vi "KeyUp.vi"(0 "Virtual Key":T1 items=["LBUTTON"=1, "RBUTTON"=2, "CANCEL"=3, "MBUTTON"=4, "BACKSPACE"=8, "TAB"=9, "CLEAR"=12, "ENTER"=13, "SHIFT"=16, "CTRL"=17, "ALT"=18, "PAUSE"=19, "CAPITAL"=20, "ESCAPE"=27, "SPACE"=32, "PAGEUP"=33, "PAGEDOWN"=34, "END"=35, "HOME"=36, "LEFTARROW"=37, "UPARROW"=38, "RIGHTARROW"=39, "DOWNARROW"=40, "SELECT"=41, "PRINT"=42, "EXECUTE"=43, "PRINTSCREEN"=44, "INSERT"=45, "DELETE"=46, "HELP"=47, "0"=48, "1"=49, "2"=50, "3"=51, "4"=52, "5"=53, "6"=54, "7"=55, "8"=56, "9"=57, "A"=65, "B"=66, "C"=67, "D"=68, "E"=69, "F"=70, "G"=71, "H"=72, "I"=73, "J"=74, "K"=75, "L"=76, "M"=77, "N"=78, "O"=79, "P"=80, "Q"=81, "R"=82, "S"=83, "T"=84, "U"=85, "V"=86, "W"=87, "X"=88, "Y"=89, "Z"=90, "LWIN"=91, "RWIN"=92, "APPS"=93, "NUMPAD0"=96, "NUMPAD1"=97, "NUMPAD2"=98, "NUMPAD3"=99, "NUMPAD4"=100, "NUMPAD5"=101, "NUMPAD6"=102, "NUMPAD7"=103, "NUMPAD8"=104, "NUMPAD9"=105, "MULTIPLY"=106, "ADD"=107, "SEPERATOR"=108, "SUBTRACT"=109, "DECIMAL"=110, "DIVIDE"=111, "F1"=112, "F2"=113, "F3"=114, "F4"=115, "F5"=116, "F6"=117, "F7"=118, "F8"=119, "F9"=120, "F10"=121, "F11"=122, "F12"=123, "F13"=124, "F14"=125, "F15"=126, "F16"=127, "F17"=128, "F18"=129, "F19"=130, "F20"=131, "F21"=132, "F22"=133, "F23"=134, "F24"=135, "NUMLOCK"=144, "SCROLL"=145, "LSHIFT"=160, "RSHIFT"=161, "LCTRL"=162, "RCTRL"=163, "LALT"=164, "RALT"=165, "VOLMUTE"=173, "VOLDOWN"=174, "VOLUP"=175, ";    :"=186, "+"=187, ",    <"=188, "_"=189, ".    >"=190, "/    ?"=191, "`    ~"=192, "[    {"=219, "\\    |"=220, "]    }"=221, "'    \""=222], 11 "error in":errorcluster) -> (15 "error out":errorcluster)   [LabVIEW 2016, in "Drona.lvlib" / "KeyboardSimulation.lvlib"]
doc: "Call the keybd_event function in user32.dll to generate an event corresponding to the key up action\nfor the desired key"
uses:
  KeyboardSimulation.lvlib
  typedef/VirtualKey.ctl
  user32.dll
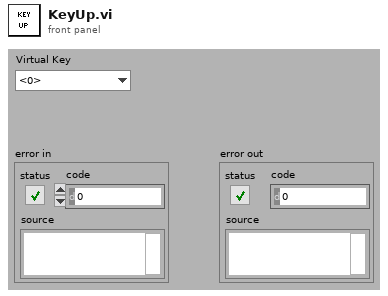
[diagram p1: front panel]
types:
  T1 = typedef "Drona.lvlib/KeyboardSimulation.lvlib/VirtualKey.ctl" = u8
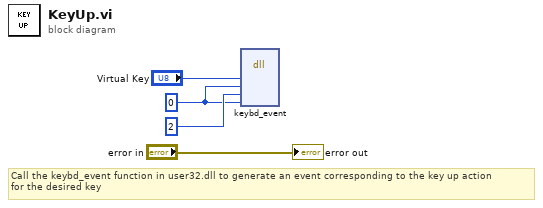
[diagram p0: block diagram]
diagram:
  w3 = u8 0 ("bScan")
  # "Call the keybd_event function in user32.dll to generate an event corresponding to the key up action\nfor the desired key"
  n1 = dll-call lib="user32.dll" fn="keybd_event"("bVk"="Virtual Key", "bScan"=w3, "dwFlags"=u32 2, "dwExtraInfo"=w3) -> ()  [unwired: 8 in, 2 out]
  "error out" <- "error in"
